vi "Create Batch Response.vi"(6 "ids":string[](array[string]), 8 "error in (no error)":errorcluster[](array[cluster]), 10 "results":variant[](array[variant]), 11 "JSON-RPC in":refnum<class "JSON-RPC.lvclass">) -> (0 "error out":errorcluster, 2 "{JSON} Response":string, 3 "JSON-RPC out":refnum<class "JSON-RPC.lvclass">)   [LabVIEW 2019, in "JSON-RPC.lvclass"]
uses:
  JSON-RPC.lvclass
  8dac1c84-94f0-4a52-a653-2d1a946a353f.vi
  8dac1c84-94f0-4a52-a653-2d1a946a353f.vi/080af00f-872a-404d-81fb-91aec086d127.vi
  8dac1c84-94f0-4a52-a653-2d1a946a353f.vi/080af00f-872a-404d-81fb-91aec086d127.vi/ddd97ab0-f880-4d62-a12b-adbfa2b80abd.vi
  8dac1c84-94f0-4a52-a653-2d1a946a353f.vi/080af00f-872a-404d-81fb-91aec086d127.vi/db6e2d89-34ae-420f-86ba-38671ee62ba9.vi
  8dac1c84-94f0-4a52-a653-2d1a946a353f.vi/080af00f-872a-404d-81fb-91aec086d127.vi/9674d577-b062-4377-a879-970cb02c3975.vi
  private/Create Error Object.vi
  <vilib>/JDP Science/JSONtext/Variant to JSON Text.vi
  <vilib>/JDP Science/JSONtext/Set Item.vi
  <vilib>/JDP Science/JSONtext/support/Format JSON Array Text.vi
  <vilib>/JDP Science/JSONtext/LVClass Serializer/JSONtext LVClass Serializer.lvclass
  <vilib>/JDP Science/JSONtext/JSONtext.lvlib
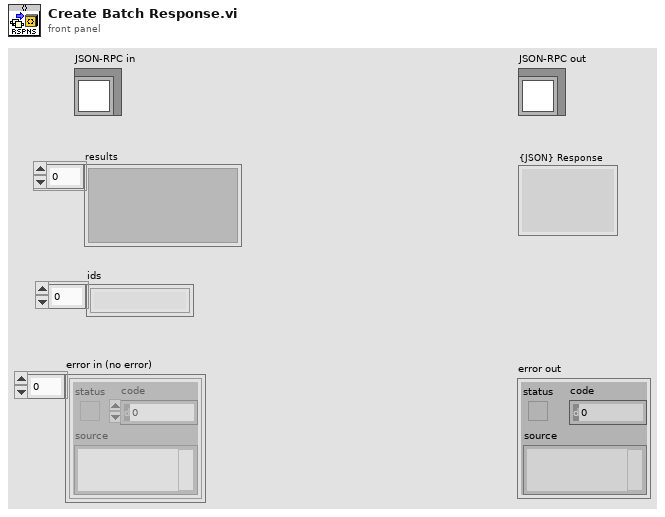
[diagram p1: front panel]
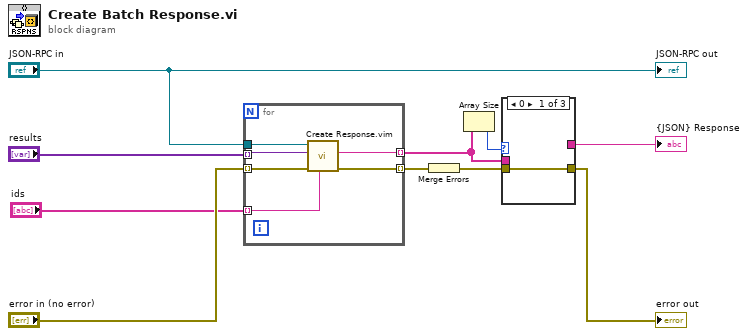
[diagram p0: block diagram]
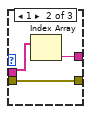
[diagram p2: hidden frame]
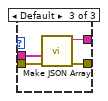
[diagram p3: hidden frame]
diagram:
  n1 = for {
    tunnel: "JSON-RPC in" -> [w16]
    tunnel: "results" -> [w15] mode=indexing
    tunnel: "error in (no error)" -> [w14] mode=indexing
    tunnel: [w13] -> w5 mode=indexing
    tunnel: [w12] -> w1 mode=indexing
    tunnel: "ids" -> [w11] mode=indexing
    n2 = call "Create Response.vim"("id"=w11, "error in (no error)"=w14, "result"=w15, "JSON-RPC in"=w16) -> ("error out"=w13:errorcluster, "{JSON} Response"=w12:string)  [unwired: 5 in, 1 out]
  }
  n3 = Merge Errors(w5) -> (w4:errorcluster)
  n4 = Array Size(array=w1) -> (size(s)=w2:i32)
  n5 = case shown="0" w2 {
    tunnel: [w17 w20 w24] -> w9
    tunnel: [_ w18 w23] -> w7
    tunnel: w4 -> [w17 w20 w22]
    tunnel: w1 -> [_ w19 w21]
    frame 0 {
    }
    frame 1 {
      n6 = Index Array(array=w19) -> (element=w18:string)  [unwired: 1 in]
    }
    frame Default {
      n7 = call <vilib>:"Make JSON Array.vi"("error in (no error)"=w22, "JSON Elements"=w21) -> ("error out"=w24:errorcluster, "<JSON>"=w23:string)  [unwired: 8 in]
    }
  }
  "error out" <- w9
  "{JSON} Response" <- w7
  "JSON-RPC out" <- "JSON-RPC in"
